vi "Main.vi"() -> ()   [LabVIEW 2018]
uses:
  State.ctl
  <vilib>/Utility/cursorutil.llb/Set Cursor (Cursor ID).vi
panel:
  out "Value":i32
  in  "Play Button":bool
  in  "Exit":bool
  in  "Button Array":bool[][](array[boolean])
  out "Display":u16[][](array[ring])
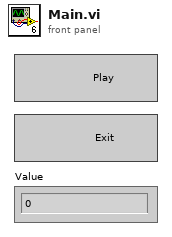
[diagram p1: front panel]
types:
  T1 = typedef "Semaphore RefNum" = refnum<k1>
  T2 = cluster{"Display Sema":T1, "vi ref":refnum<vi>[][], "Display":refnum<vi>, "Diglett Status":bool[][], "Time":timestamp[][], "Value":i32}
  T3 = typedef "State.ctl" = enum16{"Initial", "Mouse Down", "Random", "Check", "shrew Up", "shrew Down", "shrew Dead", "shrew Wrong", "Exit"}
  T4 = enum16{"Add State", "Insert State", "Initial State", "Release State", "Flush State"}
  T5 = enum16{"ªÅ¬}", "¦a¹«¤É°_", "¦a¹«¤U­°", "¦a¹«³Q¥´", "¥´¿ù¬}"}
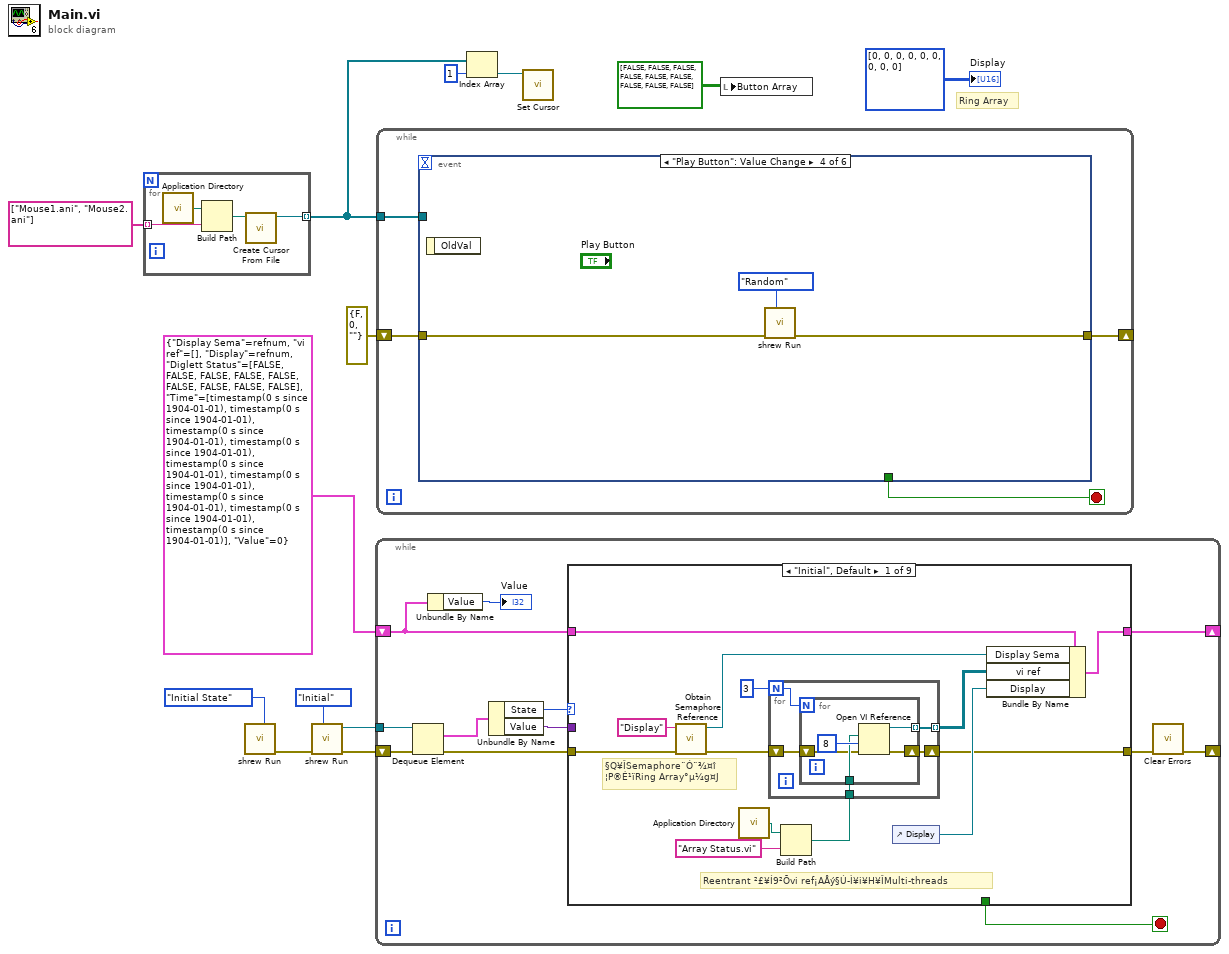
[diagram p0: block diagram]
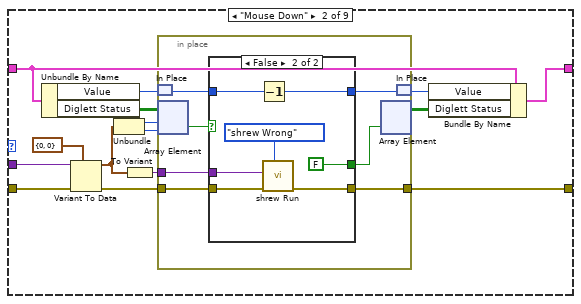
[diagram p2: hidden frame]
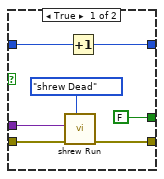
[diagram p3: hidden frame]
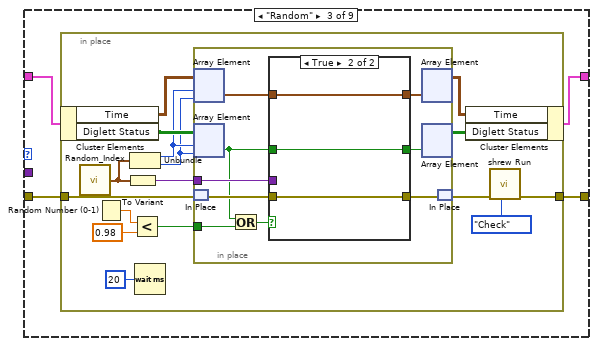
[diagram p4: hidden frame]
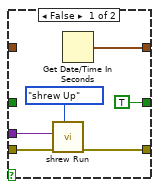
[diagram p5: hidden frame]
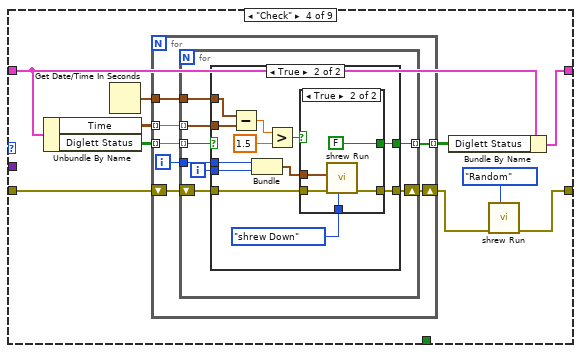
[diagram p6: hidden frame]
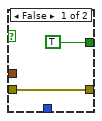
[diagram p8: hidden frame]
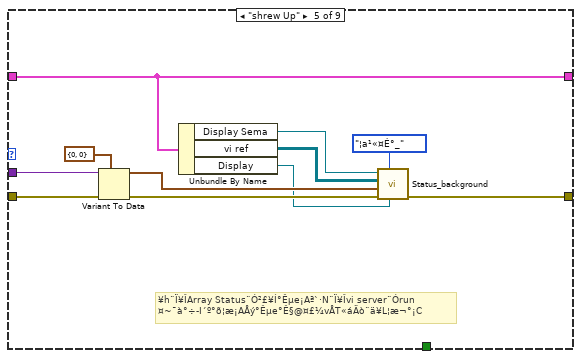
[diagram p9: hidden frame]
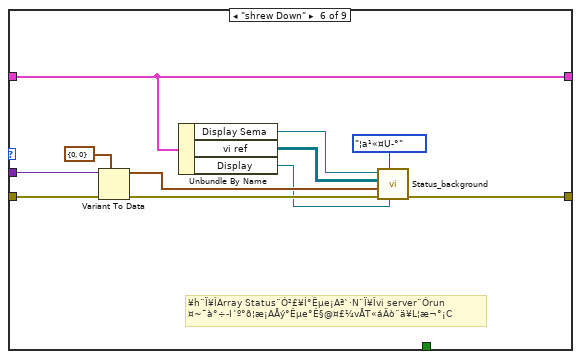
[diagram p10: hidden frame]
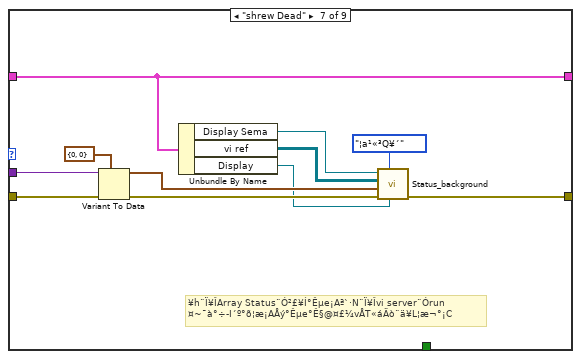
[diagram p11: hidden frame]
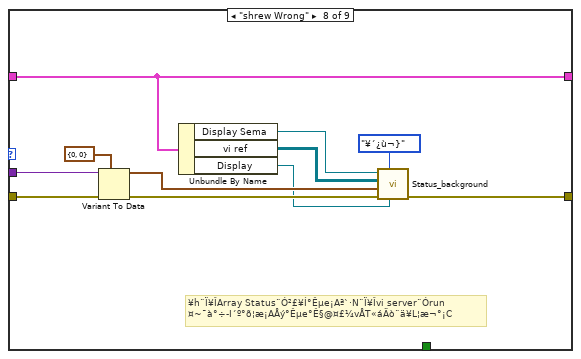
[diagram p12: hidden frame]
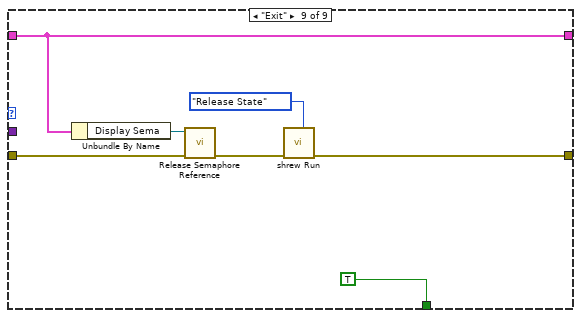
[diagram p13: hidden frame]
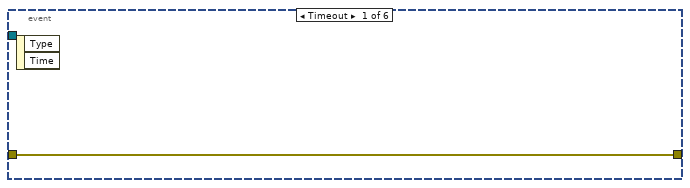
[diagram p14: hidden frame]
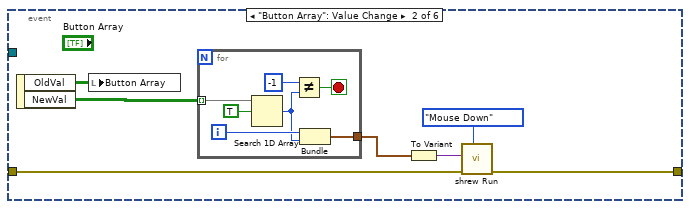
[diagram p15: hidden frame]
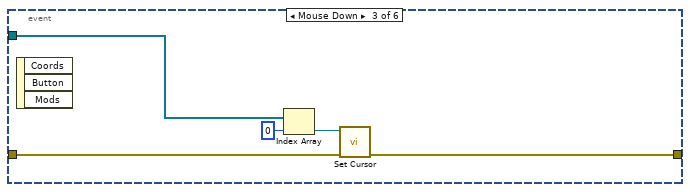
[diagram p16: hidden frame]
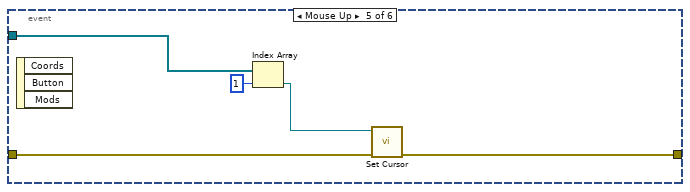
[diagram p17: hidden frame]
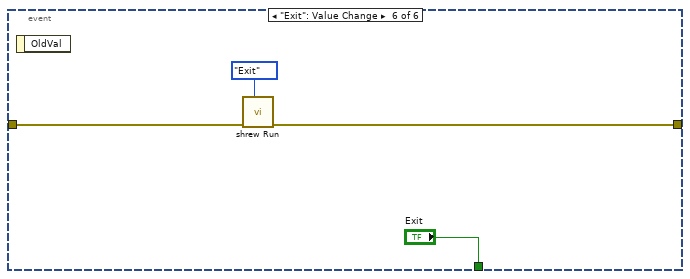
[diagram p18: hidden frame]
diagram:
  # "Ring Array"
  n1 = for {
    tunnel: [w17] -> w1 mode=indexing
    tunnel: string[] ["Mouse1.ani", "Mouse2.ani"] -> [w14] mode=indexing
    n2 = call <vilib>:"Application Directory.vi"() -> ("Application Directory"=w16:path)
    n3 = Build Path(base path=w16, name or relative path=w14) -> (appended path=w15:path)
    n4 = call <vilib>:"Create Cursor From File.vi"("cursor file"=w15) -> ("cursor ID"=w17:refnum<k1>)  [unwired: 9 in, 1 out]
  }
  n5 = call "shrew Run.vi"("Control"=T4."Initial State") -> ("error out"=w8:errorcluster)  [unwired: 9 in, 1 out]
  n6 = call "shrew Run.vi"("State"=State."Initial", "error in"=w8) -> ("error out"=w7:errorcluster, "queue out"=w11:refnum<queue>)  [unwired: 8 in]
  n7 = while {
    shift-right: [w21] -> _
    shift-left: w7 -> [w27]
    tunnel: w11 -> [w28]
    shift-right: [w20] -> _
    shift-left: T2 {"Display Sema"=refnum, "vi ref"=[], "Display"=refnum, "Diglett Status"=[[FALSE, FALSE, FALSE], [FALSE, FALSE, FALSE], [FALSE, FALSE, FALSE]], "Time"=[[timestamp(0 s since 1904-01-01), timestamp(0 s since 1904-01-01), timestamp(0 s since 1904-01-01)], [timestamp(0 s since 1904-01-01), timestamp(0 s since 1904-01-01), timestamp(0 s since 1904-01-01)], [timestamp(0 s since 1904-01-01), timestamp(0 s since 1904-01-01), timestamp(0 s since 1904-01-01)]], "Value"=0} -> [w19]
    stop <- w23 stop-if-true
    n8 = Dequeue Element(queue=w28, error in (no error)=w27) -> (element=w25:cluster{"State":T3, "Value":variant}, error out=w26:errorcluster)  [unwired: 1 in, 2 out]
    n9 = Unbundle By Name(w19) -> ("Value"=→"Value":i32)
    n10 = Unbundle By Name(w25) -> ("State"=w24:T3, "Value"=w22:variant)
    n11 = case shown="\"Initial\", Default" w24 {
      tunnel: w26 -> [w42 w67 w92 w133 w182 w193 w204 w215 w222]
      tunnel: [w30 w63 w91 w128 w178 w189 w200 w211 w217] -> w29
      tunnel: [_ _ _ _ _ _ _ _ TRUE] -> w23
      tunnel: w19 -> [w40 w58 w90 w132 w180 w191 w202 w213 w220]
      tunnel: [w38 w57 w89 w131 w180 w191 w202 w213 w220] -> w20
      tunnel: w22 -> [_ w66 _ _ w181 w192 w203 w214 _]
      frame "Initial", Default {
        # "§Q¥ÎSemaphore¨Ó¨¾¤î\n¦P®É¹ïRing Array°µ¼g¤J"
        # "Reentrant ²£¥Í9²Õvi ref¡AÅý§Ú­Ì¥i¥H¥ÎMulti-threads"
        n12 = call <vilib>:"Obtain Semaphore Reference.vi"("error in (no error)"=w42, "name (unnamed)"="Display") -> ("error out"=w33:errorcluster, "semaphore"=w39:T1)  [unwired: 3 in, 1 out]
        n13 = call <vilib>:"Application Directory.vi"() -> ("Application Directory"=w36:path)
        n14 = Build Path(base path=w36, name or relative path="Array Status.vi") -> (appended path=w37:path)
        n15 = for {
          N: 3 -> [w45]
          tunnel: [w47] -> w32 mode=indexing
          tunnel: w37 -> [w46]
          shift-right: [w44] -> w30
          shift-left: w33 -> [w43]
          n16 = for {
            N: w45 -> [_]
            tunnel: [w52] -> w47 mode=indexing
            shift-right: [w49] -> w44
            shift-left: w43 -> [w48]
            tunnel: w46 -> [w50]
            n17 = Open VI Reference(vi path=w50, options=8, error in (no error)=w48) -> (vi reference=w52:refnum<vi>, error out=w49:errorcluster)  [unwired: 3 in]
          }
        }
        n18 = control-ref of="Display"() -> (w31:refnum<vi>)
        n19 = Bundle By Name(cluster=w40, "Display Sema"=w39, "vi ref"=w32, "Display"=w31) -> (w38:T2)
      }
      frame "Mouse Down" {
        n20 = Unbundle By Name(w58) -> ("Value"=w54:i32, "Diglett Status"=w62:bool[][])
        n21 = Variant To Data(error in=w67, type=cluster{"Row":i32, "Col":i32} {"Row"=0, "Col"=0} ("Position"), Variant=w66) -> (data=w56:cluster{"Row":i32, "Col":i32}, error out=w64:errorcluster)
        n22 = Unbundle(w56) -> ("Row"=w61:i32, "Col"=w60:i32)
        n23 = To Variant(anything=w56) -> (Variant=w55:variant)
        n24 = in-place {
          in-place-border: w64 -> [w74]
          in-place-border: [w73] -> w63
          in-place-border: w55 -> [w70]
          n25 = in-place-match #1(w54) -> (w69:i32)
          n26 = in-place-array #2(w62, w61, w60) -> (w72:bool)
          n27 = case shown="False" w72 {
            tunnel: w74 -> [w80 w87]
            tunnel: [w79 w86] -> w73
            tunnel: [FALSE FALSE] -> w71
            tunnel: w70 -> [w77 w84]
            tunnel: w69 -> [w76 w83]
            tunnel: [w75 w82] -> w68
            frame True {
              n28 = call "shrew Run.vi"("State"=State."shrew Dead", "error in"=w80, "Value"=w77) -> ("error out"=w79:errorcluster)  [unwired: 7 in, 1 out]
              n29 = Increment(x=w76) -> (x+1=w75:i32)
            }
            frame False {
              n30 = Decrement(x=w83) -> (x-1=w82:i32)
              n31 = call "shrew Run.vi"("State"=State."shrew Wrong", "error in"=w87, "Value"=w84) -> ("error out"=w86:errorcluster)  [unwired: 7 in, 1 out]
            }
          }
          n32 = in-place-array #2(w71) -> (w59:bool[][])  [unwired: 2 out]
          n33 = in-place-match #1(w68) -> (w53:i32)
        }
        n34 = Bundle By Name(cluster=w58, "Value"=w53, "Diglett Status"=w59) -> (w57:T2)
      }
      frame "Random" {
        n35 = in-place {
          in-place-border: w92 -> [w108]
          in-place-border: [w94] -> w91
          n36 = in-place-cluster #3(w90) -> ("Time"=w105:timestamp[][], "Diglett Status"=w107:bool[][])
          n37 = call "Random_Index.vi"() -> ("Position"=w104:cluster{"Row":i32, "Col":i32})
          n38 = Random Number (0-1)() -> (number: 0 to 1=w100:dbl)
          n39 = To Variant(anything=w104) -> (Variant=w99:variant)
          n40 = Unbundle(w104) -> ("Row"=w103:i32, "Col"=w102:i32)
          n41 = Less?(x=w100, y=0.98) -> (x < y?=w98:bool)
          n42 = Wait (ms)(milliseconds to wait=u32 20) -> ()  [unwired: 1 out]
          n43 = in-place {
            in-place-border: w99 -> [w114]
            in-place-border: w98 -> [w112]
            n44 = in-place-array #4(w105, w103, w102) -> (w109:timestamp)
            n45 = in-place-array #5(w107, w103, w102) -> (w111:bool)
            n46 = in-place-match #6(w108) -> (w116:errorcluster)
            n47 = Or(x=w111, y=w112) -> (x .or. y?=w113:bool)
            n48 = case shown="True" w113 {
              tunnel: [TRUE w125] -> w117
              tunnel: w116 -> [w121 w126]
              tunnel: w114 -> [w120 _]
              tunnel: [w119 w126] -> w115
              tunnel: w111 -> [_ w125]
              tunnel: [w118 w124] -> w110
              tunnel: w109 -> [_ w124]
              frame False {
                n49 = call "shrew Run.vi"("State"=State."shrew Up", "error in"=w121, "Value"=w120) -> ("error out"=w119:errorcluster)  [unwired: 7 in, 1 out]
                n50 = Get Date/Time In Seconds() -> (seconds since 1Jan1904=w118:timestamp)
              }
              frame True {
              }
            }
            n51 = in-place-array #4(w110) -> (w93:timestamp[][])  [unwired: 2 out]
            n52 = in-place-array #5(w117) -> (w106:bool[][])  [unwired: 2 out]
            n53 = in-place-match #6(w115) -> (w95:errorcluster)
          }
          n54 = in-place-cluster #3("Time"=w93, "Diglett Status"=w106) -> (w89:T2)
          n55 = call "shrew Run.vi"("State"=State."Check", "error in"=w95) -> ("error out"=w94:errorcluster)  [unwired: 8 in, 1 out]
        }
      }
      frame "Check" {
        n56 = Unbundle By Name(w132) -> ("Time"=w136:timestamp[][], "Diglett Status"=w135:bool[][])
        n57 = Get Date/Time In Seconds() -> (seconds since 1Jan1904=w134:timestamp)
        n58 = for {
          tunnel: w136 -> [w143] mode=indexing
          tunnel: w135 -> [w142] mode=indexing
          tunnel: w134 -> [w141]
          tunnel: [w140] -> w127 mode=indexing
          shift-right: [w137] -> w129
          shift-left: w133 -> [w138]
          i -> [w139]
          n59 = for {
            tunnel: w143 -> [w151] mode=indexing
            tunnel: w142 -> [w149] mode=indexing
            tunnel: w141 -> [w150]
            tunnel: [w148] -> w140 mode=indexing
            tunnel: w139 -> [w147]
            shift-right: [w145] -> w137
            shift-left: w138 -> [w146]
            i -> [w144]
            n60 = case shown="True" w149 {
              selector: w149 -> [w153 _]
              tunnel: w151 -> [_ w165]
              tunnel: w150 -> [_ w164]
              tunnel: [w153 w159] -> w148
              tunnel: w147 -> [_ w161]
              tunnel: w146 -> [w152 w158]
              tunnel: [w152 w157] -> w145
              tunnel: w144 -> [_ w156]
              frame False {
              }
              frame True {
                n61 = Subtract(x=w164, y=w165) -> (x-y=w163:dbl)
                n62 = Bundle(w161, w156) -> (w154:cluster{i32, i32})  [unwired: 1 in]
                n63 = Greater?(x=w163, y=1.5) -> (0:w160:bool)
                n64 = case shown="True" w160 {
                  tunnel: [TRUE FALSE] -> w159
                  tunnel: w158 -> [w167 w171]
                  tunnel: [w167 w170] -> w157
                  tunnel: State."shrew Down" ("State") -> [_ w169]
                  tunnel: w154 -> [_ w168]
                  frame False {
                  }
                  frame True {
                    n65 = call "shrew Run.vi"("State"=w169, "error in"=w171, "Value"=w168) -> ("error out"=w170:errorcluster)  [unwired: 7 in, 1 out]
                  }
                }
              }
            }
          }
        }
        n66 = Bundle By Name(cluster=w132, "Diglett Status"=w127) -> (w131:T2)
        n67 = call "shrew Run.vi"("State"=State."Random", "error in"=w129) -> ("error out"=w128:errorcluster)  [unwired: 8 in, 1 out]
      }
      frame "shrew Up" {
        # "¥h¨Ï¥ÎArray Status¨Ó²£¥Í°Êµe¡Aª`·N¨Ï¥Îvi server¨Órun\n¤~¯à°÷­I´º°õ¦æ¡AÅý°Êµe°Ê§@¤£¼vÅT«áÄò¨ä¥L¦æ¬°¡C"
        n68 = Variant To Data(error in=w182, type=cluster{"Row":i32, "Col":i32} {"Row"=0, "Col"=0} ("Position"), Variant=w181) -> (data=w175:cluster{"Row":i32, "Col":i32}, error out=w179:errorcluster)
        n69 = Unbundle By Name(w180) -> ("Display Sema"=w176:T1, "vi ref"=w177:refnum<vi>[][], "Display"=w173:refnum<vi>)
        n70 = call "Status_background.vi"("Display"=w173, "Action"=T5."¦a¹«¤É°_", "error in (no error)"=w179, "Position"=w175, "vi ref"=w177, "Display Sema"=w176) -> ("error out"=w178:errorcluster)  [unwired: 5 in]
      }
      frame "shrew Down" {
        # "¥h¨Ï¥ÎArray Status¨Ó²£¥Í°Êµe¡Aª`·N¨Ï¥Îvi server¨Órun\n¤~¯à°÷­I´º°õ¦æ¡AÅý°Êµe°Ê§@¤£¼vÅT«áÄò¨ä¥L¦æ¬°¡C"
        n71 = Variant To Data(error in=w193, type=cluster{"Row":i32, "Col":i32} {"Row"=0, "Col"=0} ("Position"), Variant=w192) -> (data=w186:cluster{"Row":i32, "Col":i32}, error out=w190:errorcluster)
        n72 = Unbundle By Name(w191) -> ("Display Sema"=w187:T1, "vi ref"=w188:refnum<vi>[][], "Display"=w184:refnum<vi>)
        n73 = call "Status_background.vi"("Display"=w184, "Action"=T5."¦a¹«¤U­°", "error in (no error)"=w190, "Position"=w186, "vi ref"=w188, "Display Sema"=w187) -> ("error out"=w189:errorcluster)  [unwired: 5 in]
      }
      frame "shrew Dead" {
        # "¥h¨Ï¥ÎArray Status¨Ó²£¥Í°Êµe¡Aª`·N¨Ï¥Îvi server¨Órun\n¤~¯à°÷­I´º°õ¦æ¡AÅý°Êµe°Ê§@¤£¼vÅT«áÄò¨ä¥L¦æ¬°¡C"
        n74 = Variant To Data(error in=w204, type=cluster{"Row":i32, "Col":i32} {"Row"=0, "Col"=0} ("Position"), Variant=w203) -> (data=w197:cluster{"Row":i32, "Col":i32}, error out=w201:errorcluster)
        n75 = Unbundle By Name(w202) -> ("Display Sema"=w198:T1, "vi ref"=w199:refnum<vi>[][], "Display"=w195:refnum<vi>)
        n76 = call "Status_background.vi"("Display"=w195, "Action"=T5."¦a¹«³Q¥´", "error in (no error)"=w201, "Position"=w197, "vi ref"=w199, "Display Sema"=w198) -> ("error out"=w200:errorcluster)  [unwired: 5 in]
      }
      frame "shrew Wrong" {
        # "¥h¨Ï¥ÎArray Status¨Ó²£¥Í°Êµe¡Aª`·N¨Ï¥Îvi server¨Órun\n¤~¯à°÷­I´º°õ¦æ¡AÅý°Êµe°Ê§@¤£¼vÅT«áÄò¨ä¥L¦æ¬°¡C"
        n77 = Variant To Data(error in=w215, type=cluster{"Row":i32, "Col":i32} {"Row"=0, "Col"=0} ("Position"), Variant=w214) -> (data=w208:cluster{"Row":i32, "Col":i32}, error out=w212:errorcluster)
        n78 = Unbundle By Name(w213) -> ("Display Sema"=w209:T1, "vi ref"=w210:refnum<vi>[][], "Display"=w206:refnum<vi>)
        n79 = call "Status_background.vi"("Display"=w206, "Action"=T5."¥´¿ù¬}", "error in (no error)"=w212, "Position"=w208, "vi ref"=w210, "Display Sema"=w209) -> ("error out"=w211:errorcluster)  [unwired: 5 in]
      }
      frame "Exit" {
        n80 = Unbundle By Name(w220) -> ("Display Sema"=w221:T1)
        n81 = call <vilib>:"Release Semaphore Reference.vi"("error in (no error)"=w222, "semaphore"=w221) -> ("error out"=w218:errorcluster)  [unwired: 8 in, 1 out]
        n82 = call "shrew Run.vi"("Control"=T4."Release State", "error in"=w218) -> ("error out"=w217:errorcluster)  [unwired: 8 in, 1 out]
      }
    }
    n83 = call <vilib>:"Clear Errors.vi"("error in (no error)"=w29) -> ("error out"=w21:errorcluster)  [unwired: 5 in, 1 out]
  }
  n84 = while {
    shift-right: [w226] -> _
    shift-left: errorcluster {"status"=FALSE, "code"=0, "source"=""} ("error out") -> [w227]
    tunnel: w1 -> [w224]
    stop <- w225 stop-if-true
    n85 = event shown="[3] \"Play Button\": Value Change" {
      selector: _ -> [_ _ _ _ _ _]
      dyn-events: _ -> [_ _ _ _ _ _]
      timeout: _ -> [_ _ _ _ _ _]
      tunnel: w227 -> [w228 w232 w245 w249 w253 w257]
      tunnel: [w228 w229 w244 w248 w252 w258] -> w226
      tunnel: [_ _ _ _ _ "Exit"] -> w225
      tunnel: w224 -> [_ _ w243 _ w251 _]
      event Timeout {
        n86 = event-data() -> ()  [unwired: 1 in, 2 out]
      }
      event "Button Array": Value Change {
        n87 = event-data() -> ("OldVal"=w234:bool[][], "NewVal"=w235:bool[][])  [unwired: 1 in]
        n88 = local write "Button Array"(w234) -> ()
        n89 = for {
          tunnel: w235 -> [w242] mode=indexing
          tunnel: [w236] -> w231
          i -> [w238]
          stop <- w239 stop-if-true
          n90 = Search 1D Array(1D array=w242, element=TRUE) -> (index of element=w237:i32)  [unwired: 1 in]
          n91 = Not Equal?(x=-1, y=w237) -> (x != y?=w239:bool)
          n92 = Bundle(w238, "index of element"=w237) -> (w236:cluster{i32, "index of element":i32})  [unwired: 1 in]
        }
        n93 = To Variant(anything=w231) -> (Variant=w230:variant)
        n94 = call "shrew Run.vi"("State"=State."Mouse Down", "error in"=w232, "Value"=w230) -> ("error out"=w229:errorcluster)  [unwired: 7 in, 1 out]
      }
      event Mouse Down {
        n95 = event-data() -> ()  [unwired: 1 in, 3 out]
        n96 = Index Array(array=w243, index=0) -> (element=w246:refnum<k1>)
        n97 = call-poly <vilib>:"Set Cursor.vi"("error in (no error)"=w245, "cursor ID"=w246) -> ("error out"=w244:errorcluster)  [unwired: 8 in, 1 out]
      }
      event "Play Button": Value Change {
        n98 = event-data() -> ()  [unwired: 1 in, 1 out]
        n99 = call "shrew Run.vi"("State"=State."Random", "error in"=w249) -> ("error out"=w248:errorcluster)  [unwired: 8 in, 1 out]
      }
      event Mouse Up {
        n100 = event-data() -> ()  [unwired: 1 in, 3 out]
        n101 = Index Array(array=w251, index=1) -> (element=w254:refnum<k1>)
        n102 = call-poly <vilib>:"Set Cursor.vi"("error in (no error)"=w253, "cursor ID"=w254) -> ("error out"=w252:errorcluster)  [unwired: 8 in, 1 out]
      }
      event "Exit": Value Change {
        n103 = event-data() -> ()  [unwired: 1 in, 1 out]
        n104 = call "shrew Run.vi"("State"=State."Exit", "error in"=w257) -> ("error out"=w258:errorcluster)  [unwired: 8 in, 1 out]
      }
    }
  }
  n105 = Index Array(array=w1, index=1) -> (element=w3:refnum<k1>)
  n106 = call-poly <vilib>:"Set Cursor.vi"("cursor ID"=w3) -> ()  [unwired: 9 in, 2 out]
  n107 = local write "Button Array"(bool[][] [[FALSE, FALSE, FALSE], [FALSE, FALSE, FALSE], [FALSE, FALSE, FALSE]] ("Button Array")) -> ()
  "Display" <- u16[][] [[0, 0, 0], [0, 0, 0], [0, 0, 0]] ("Display")
